vi "GEOM_UpdateDetInfo.vi"(8 "error in (no error)":errorcluster, 9 "section":string="INFO", 10 "Info In":string[][](table), 11 "configuration file path":path=path "/home/ArcVIEW/Modules/Geometry/database/TYPES/Hawaii-II_4ch.chp") -> (0 "error out":errorcluster, 2 "Info Out":string[][](table), 3 "file path out":path=path "/home/ArcVIEW/Modules/Geometry/database/TYPES/Hawaii-II_4ch.chp")   [LabVIEW 2016]
uses:
  <vilib>/Utility/config.llb/Read Key (String).vi
  <vilib>/Utility/config.llb/NI_LVConfig.lvlib
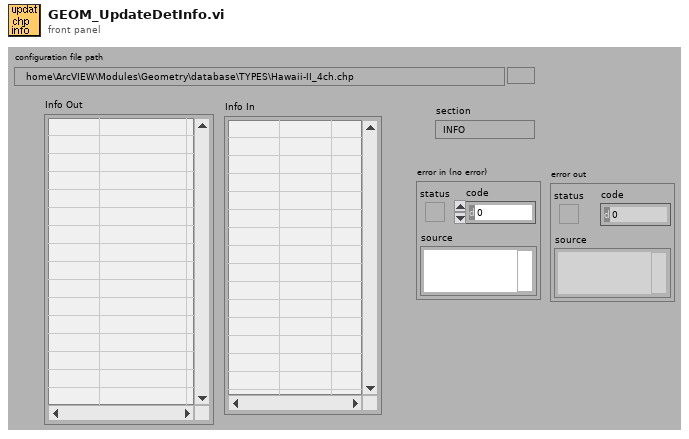
[diagram p1: front panel]
types:
  T1 = typedef "NI_LVConfig.lvlib/Config Data RefNum.ctl" = refnum<k1>
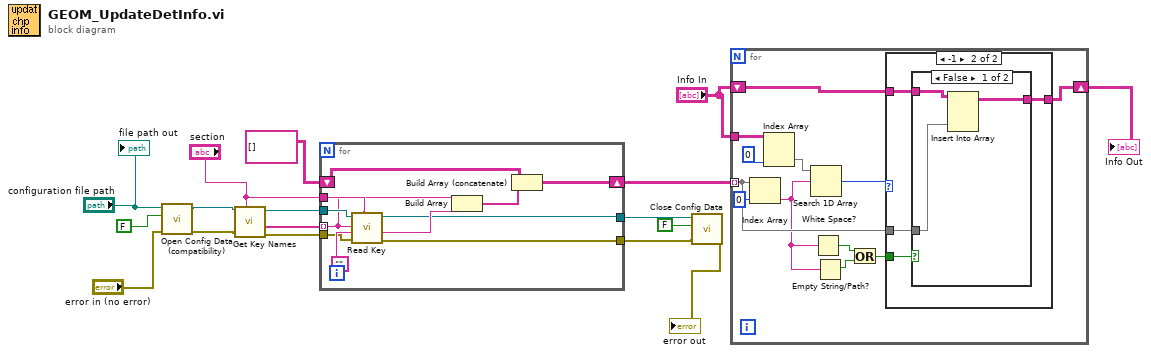
[diagram p0: block diagram]
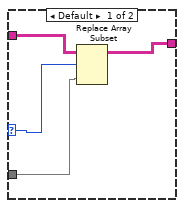
[diagram p2: hidden frame]
diagram:
  n1 = call <vilib>:"Open Config Data (compatibility).vi"("error in (no error)"="error in (no error)", "create file if necessary (T)"=FALSE ("create file if necessary? (T)"), "configuration file path"="configuration file path") -> ("error out"=w15:errorcluster, "refnum"=w16:T1)  [unwired: 6 in, 1 out]
  n2 = call <vilib>:"Get Key Names.vi"("section"="section", "error in (no error)"=w15, "refnum"=w16) -> ("error out"=w9:errorcluster, "key names"=w14:string[], "refnum out"=w12:T1)  [unwired: 6 out]
  n3 = for {
    tunnel: w14 -> [w25] mode=indexing
    tunnel: "section" -> [w28]
    tunnel: w12 -> [w27]
    shift-right: [w22] -> w6
    shift-left: string[][] [] -> [w21]
    tunnel: [w20] -> w10
    tunnel: w9 -> [w19]
    tunnel: [w18] -> w8
    n4 = call-poly <vilib>:"Read Key.vi"("section"=w28, "error in (no error)"=w19, "default value"="", "key"=w25, "refnum"=w27) -> ("error out"=w18:errorcluster, "value"=w24:string, "refnum out"=w20:T1)  [unwired: 1 in, 3 out]
    n5 = Build Array(w25, w24) -> (w23:string[])
    n6 = Build Array (concatenate)(w21, w23) -> (w22:string[][])
  }
  n7 = call <vilib>:"Close Config Data.vi"("error in (no error)"=w8, "write file if changed (T)"=FALSE ("write configuration file? (F)"), "refnum"=w10) -> ("error out"=→"error out":errorcluster)  [unwired: 8 out]
  n8 = for {
    tunnel: w6 -> [w35] mode=indexing
    tunnel: "Info In" -> [w39]
    shift-right: [w34] -> w4
    shift-left: "Info In" -> [w36]
    n9 = Index Array(array=w35, index=0) -> (element=w33:string)
    n10 = Index Array(array=w39, index (col)=0 ("index")) -> (element=w38:string[])  [unwired: 1 in]
    n11 = Search 1D Array(1D array=w38, element=w33) -> (index of element=w30:i32)  [unwired: 1 out]
    n12 = White Space?(1:w33) -> (0:w32:bool)
    n13 = Empty String/Path?(string/path=w33) -> (empty?=w31:bool)
    n14 = Or(x=w32, y=w31) -> (x .or. y?=w29:bool)
    n15 = case shown="-1" w30 {
      selector: w30 -> [w42 _]
      tunnel: w36 -> [w44 w48]
      tunnel: w35 -> [w43 w47]
      tunnel: [w41 w46] -> w34
      tunnel: w29 -> [_ w45]
      frame Default {
        n16 = Replace Array Subset(array=w44, new element=w43, index (row)=w42) -> (w41:string[][])  [unwired: 1 in]
      }
      frame -1 {
        n17 = case shown="False" w45 {
          tunnel: w48 -> [w51 w52]
          tunnel: w47 -> [w50 _]
          tunnel: [w49 w52] -> w46
          frame False {
            n18 = Insert Into Array(array=w51, new element=w50) -> (w49:string[][])  [unwired: 2 in]
          }
          frame True {
          }
        }
      }
    }
  }
  "Info Out" <- w4
  "file path out" <- "configuration file path"
